vi "FGV_AnalysersControl.vi"(6 "String Input":string, 7 "Action":T2=enum."Get ID", 8 "Error In":errorcluster, 9 "Set Voltage":dbl, 10 "Analyser":i32=1 min=1 max=2 step=1, 11 "VISA resource In":refnum<visa-resource-name>) -> (0 "error out":errorcluster, 2 "Received":string, 3 "VISA resource Out":refnum<visa-resource-name>)   [LabVIEW 2014]
uses:
  TypeDef_AnalyserActions.ctl
panel:
  out "Use Checksum":bool
  in  "Maximum Voltages":T1={"RE"=300.0, "LE"=100.0, "DX"=11.0, "DY"=11.0, "AM"=15.0, "IH"=35.0, "OH"=20.0}
  in  "Minimum Voltages":T1={"RE"=0.0, "LE"=0.0, "DX"=-11.0, "DY"=-11.0, "AM"=0.0, "IH"=5.0, "OH"=5.0}
  # "To update calibration, change the values above\nBE SURE TO CLICK EDIT->MAKE CURRENT VALUES DEFAULT"
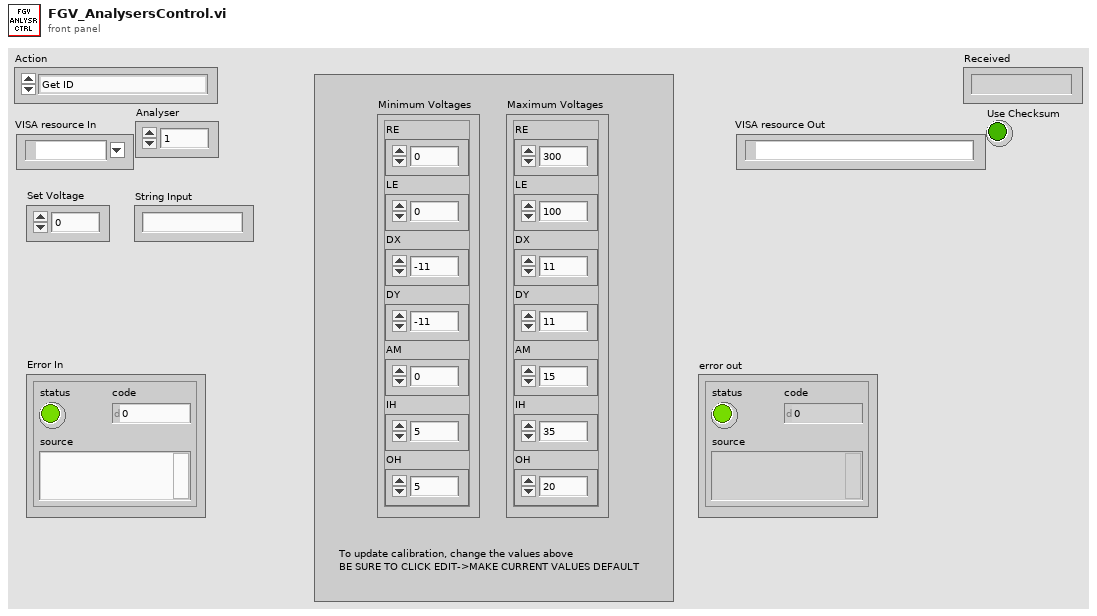
[diagram p1: front panel]
types:
  T1 = cluster{"RE":dbl, "LE":dbl, "DX":dbl, "DY":dbl, "AM":dbl, "IH":dbl, "OH":dbl}
  T2 = typedef "TypeDef_AnalyserActions.ctl" = enum16{"Find COM Port", "Find & Connect", "Connect Port", "Disconnect Port", "Enable Checksum", "Disable Checksum", "Get ID", "Msg & ACKNAK", "Msg & Response", "Set RE Voltage", "Set LE Voltage", "Set DX Voltage", "Set DY Voltage", "Set AM Voltage", "Set IH Voltage", "Set OH Voltage", "Get AE", "Get RE", "Get LE", "Get DX", "Get DY", "Get AM", "Get IH", "Get OH"}
  T3 = cluster{"Maximum Voltages":cluster{"RE":dbl, "LE":dbl, "DX":dbl, "DY":dbl, "AM":dbl, "IH":dbl, "OH":dbl}, "Minimum Voltages":cluster{"RE":dbl, "LE":dbl, "DX":dbl, "DY":dbl, "AM":dbl, "IH":dbl, "OH":dbl}}
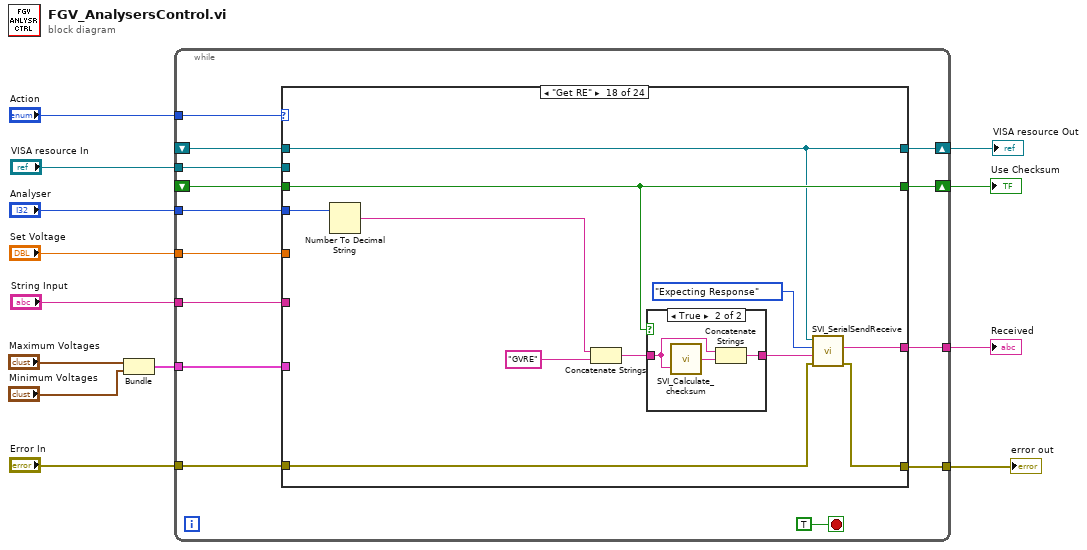
[diagram p0: block diagram]
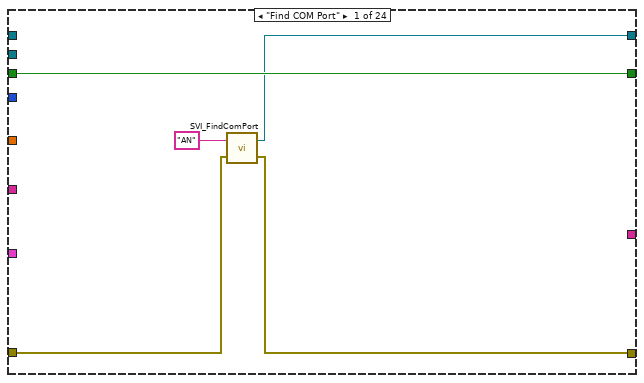
[diagram p2: hidden frame]
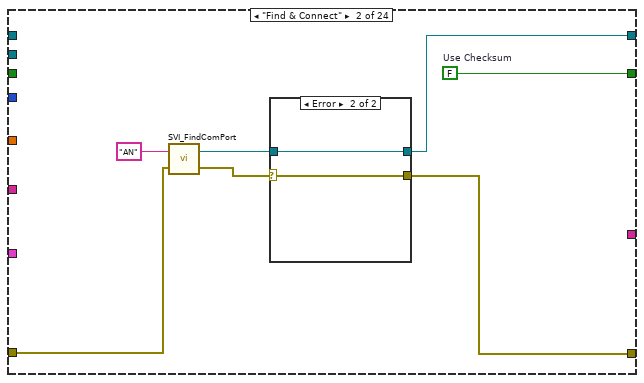
[diagram p3: hidden frame]
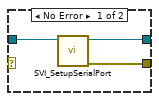
[diagram p4: hidden frame]
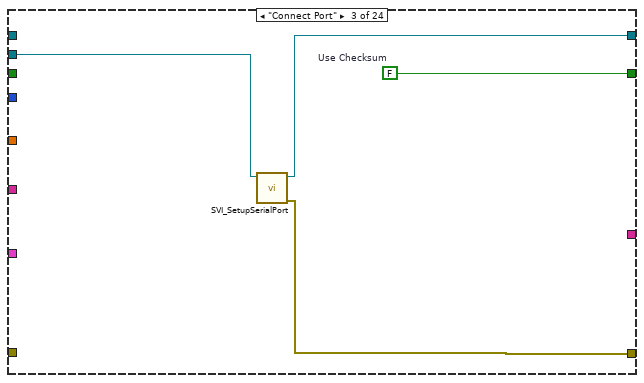
[diagram p5: hidden frame]
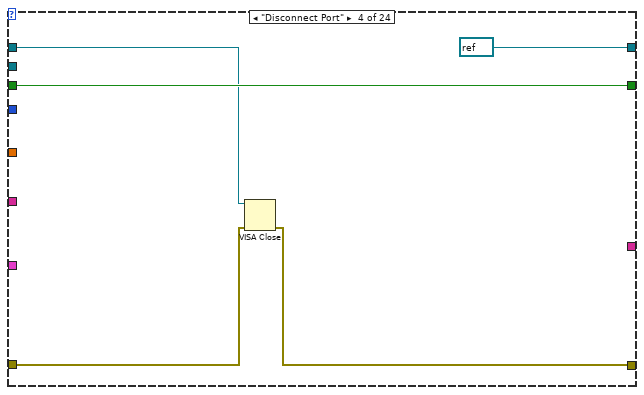
[diagram p6: hidden frame]
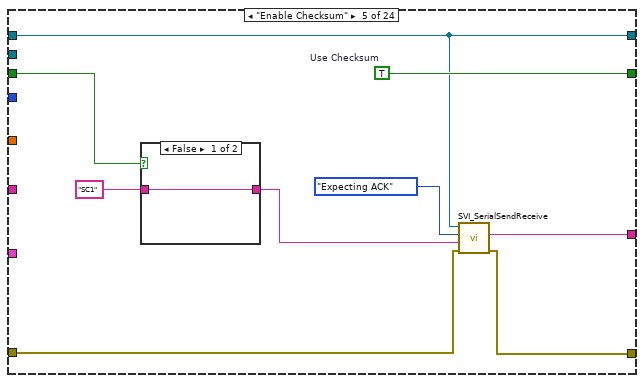
[diagram p7: hidden frame]
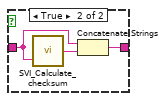
[diagram p8: hidden frame]
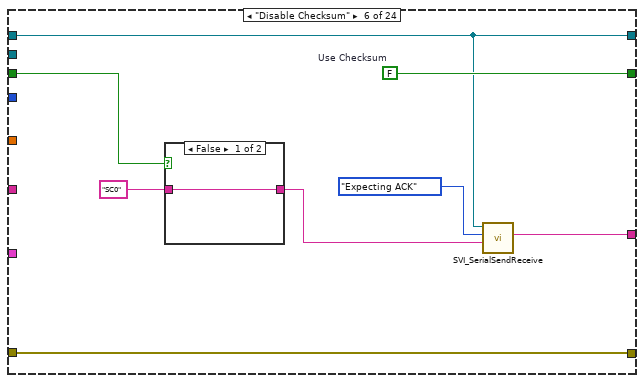
[diagram p9: hidden frame]
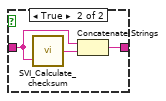
[diagram p10: hidden frame]
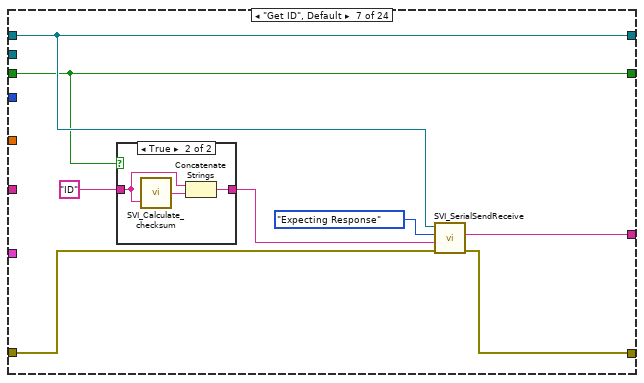
[diagram p11: hidden frame]
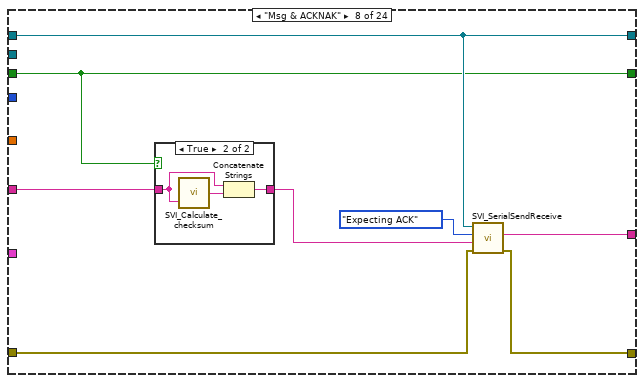
[diagram p13: hidden frame]
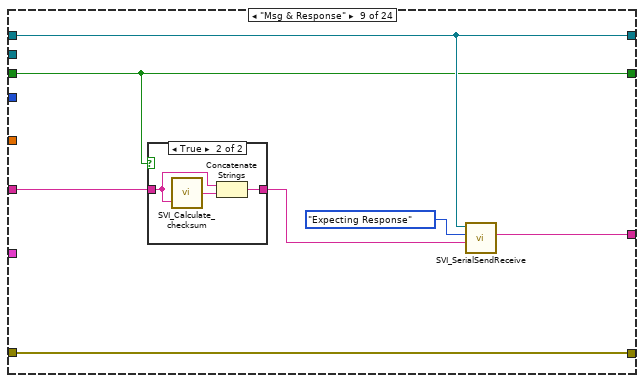
[diagram p15: hidden frame]
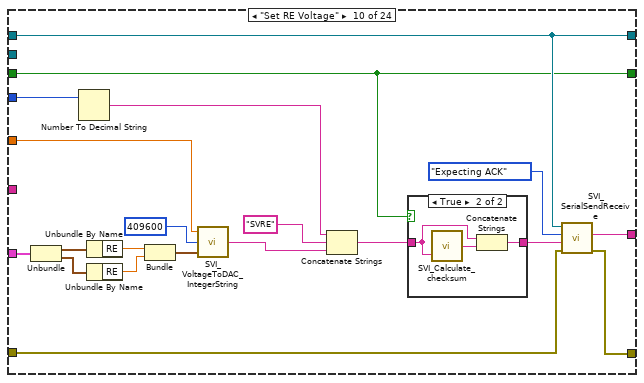
[diagram p17: hidden frame]
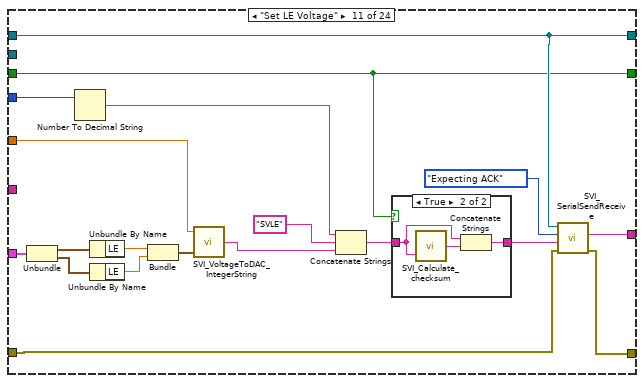
[diagram p19: hidden frame]
diagram:
  n1 = Bundle("Maximum Voltages"="Maximum Voltages", "Minimum Voltages"="Minimum Voltages") -> (w2:T3)  [unwired: 1 in]
  n2 = while {
    tunnel: "Action" -> [w26]
    tunnel: "VISA resource In" -> [w25]
    shift-right: [w24] -> w11
    shift-left: _ -> [w23]
    tunnel: "Error In" -> [w22]
    tunnel: [w21] -> w9
    tunnel: w2 -> [w20]
    tunnel: "Set Voltage" -> [w19]
    shift-right: [w18] -> w6
    shift-left: _ -> [w17]
    tunnel: "String Input" -> [w16]
    tunnel: [w15] -> w7
    tunnel: "Analyser" -> [w14]
    stop <- TRUE stop-if-true
    n3 = case shown="\"Get RE\"" w26 {
      tunnel: w25 -> [_ _ w46 _ _ _ _ _ _ _ _ _ _ _ _ _ _ _ _ _ _ _ _ _]
      tunnel: [w30 w33 w45 refnum<visa-resource-name> refnum ("VISA Refnum out") w57 w67 w83 w95 w105 w130 w147 w163 w188 w213 w230 w254 w279 w293 w306 w324 w338 w353 w369 w381] -> w24
      tunnel: w23 -> [_ _ _ w50 w57 w67 w83 w95 w105 w130 w147 w163 w188 w213 w230 w254 w279 w293 w306 w324 w338 w353 w369 w381]
      tunnel: [w28 w34 w47 w51 w55 w74 w84 w94 w109 w128 w145 w165 w187 w208 w236 w256 w278 w292 w309 w322 w339 w354 w367 w384] -> w21
      tunnel: w22 -> [w29 w37 _ w52 w56 w74 w85 w93 w109 w129 w144 w164 w186 w207 w235 w255 w277 w291 w308 w321 w340 w355 w366 w383]
      tunnel: w20 -> [_ _ _ _ _ _ _ _ _ w121 w149 w166 w184 w211 w234 w258 _ _ _ _ _ _ _ _]
      tunnel: w19 -> [_ _ _ _ _ _ _ _ _ w127 w148 w167 w191 w210 w233 w260 _ _ _ _ _ _ _ _]
      tunnel: [w32 w39 w48 w53 w62 w73 w80 w92 w103 w119 w143 w162 w189 w214 w231 w253 w280 w294 w307 w325 w337 w352 w370 w385] -> w18
      tunnel: w17 -> [w32 _ _ w53 w58 w68 w80 w92 w103 w119 w143 w162 w189 w214 w231 w253 w280 w294 w307 w325 w337 w352 w370 w385]
      tunnel: w16 -> [_ _ _ _ _ _ _ w91 w104 _ _ _ _ _ _ _ _ _ _ _ _ _ _ _]
      tunnel: [_ _ _ _ w54 w69 w79 w96 w106 w131 w146 w161 w185 w212 w237 w257 w276 w296 w310 w323 w341 w356 w368 w382] -> w15
      tunnel: w14 -> [_ _ _ _ _ _ _ _ _ w118 w142 w168 w190 w209 w232 w259 w281 w295 w311 w326 w336 w351 w371 w386]
      frame "Find COM Port" {
        n4 = call "SVI_FindComPort.vi"("Error In"=w29, "ID to Match"="AN") -> ("error out"=w28:errorcluster, "VISA resource name"=w30:refnum<visa-resource-name>)
      }
      frame "Find & Connect" {
        w39 = FALSE  # Use Checksum
        n5 = call "SVI_FindComPort.vi"("Error In"=w37, "ID to Match"="AN") -> ("error out"=w36:errorcluster, "VISA resource name"=w35:refnum<visa-resource-name>)
        n6 = case shown="Error" w36 {
          selector: w36 -> [_ w44]
          tunnel: w35 -> [w42 w43]
          tunnel: [w41 w44] -> w34
          tunnel: [w40 w43] -> w33
          frame No Error {
            n7 = call "SVI_SetupSerialPort.vi"("VISA Refnum in"=w42) -> ("error out"=w41:errorcluster, "VISA Refnum out"=w40:refnum<visa-resource-name>)  [unwired: 9 in]
          }
          frame Error {
          }
        }
      }
      frame "Connect Port" {
        w48 = FALSE  # Use Checksum
        n8 = call "SVI_SetupSerialPort.vi"("VISA Refnum in"=w46) -> ("error out"=w47:errorcluster, "VISA Refnum out"=w45:refnum<visa-resource-name>)  [unwired: 9 in]
      }
      frame "Disconnect Port" {
        n9 = VISA Close(VISA resource name=w50, error in (no error)=w52) -> (error out=w51:errorcluster)
      }
      frame "Enable Checksum" {
        w62 = TRUE  # Use Checksum
        n10 = case shown="False" w58 {
          tunnel: "SC1" ("write buffer") -> [w63 w64]
          tunnel: [w63 w65] -> w60
          frame False {
          }
          frame True {
            n11 = call "SVI_Calculate_checksum.vi"("Message"=w64) -> ("Calculated checksum"=w66:string)  [unwired: 1 in]
            n12 = Concatenate Strings(w64, w66) -> (w65:string)
          }
        }
        n13 = call "SVI_SerialSendReceive.vi"("error in (no error)"=w56, "Command"=w60, "Message Type"=enum16{"Expecting Response", "Expecting ACK"}."Expecting ACK", "VISA Refnum in"=w57) -> ("error out"=w55:errorcluster, "Received"=w54:string)  [unwired: 4 in, 2 out]
      }
      frame "Disable Checksum" {
        w73 = FALSE  # Use Checksum
        n14 = case shown="False" w68 {
          tunnel: "SC0" ("write buffer") -> [w75 w76]
          tunnel: [w75 w77] -> w71
          frame False {
          }
          frame True {
            n15 = call "SVI_Calculate_checksum.vi"("Message"=w76) -> ("Calculated checksum"=w78:string)  [unwired: 1 in]
            n16 = Concatenate Strings(w76, w78) -> (w77:string)
          }
        }
        n17 = call "SVI_SerialSendReceive.vi"("Command"=w71, "Message Type"=enum16{"Expecting Response", "Expecting ACK"}."Expecting ACK", "VISA Refnum in"=w67) -> ("Received"=w69:string)  [unwired: 5 in, 3 out]
      }
      frame "Get ID", Default {
        n18 = case shown="True" w80 {
          tunnel: "ID" ("write buffer") -> [w87 w88]
          tunnel: [w87 w89] -> w82
          frame False {
          }
          frame True {
            n19 = call "SVI_Calculate_checksum.vi"("Message"=w88) -> ("Calculated checksum"=w90:string)  [unwired: 1 in]
            n20 = Concatenate Strings(w88, w90) -> (w89:string)
          }
        }
        n21 = call "SVI_SerialSendReceive.vi"("error in (no error)"=w85, "Command"=w82, "Message Type"=enum16{"Expecting Response", "Expecting ACK"}."Expecting Response", "VISA Refnum in"=w83) -> ("error out"=w84:errorcluster, "Received"=w79:string)  [unwired: 4 in, 2 out]
      }
      frame "Msg & ACKNAK" {
        n22 = case shown="True" w92 {
          tunnel: w91 -> [w99 w100]
          tunnel: [w99 w101] -> w98
          frame False {
          }
          frame True {
            n23 = call "SVI_Calculate_checksum.vi"("Message"=w100) -> ("Calculated checksum"=w102:string)  [unwired: 1 in]
            n24 = Concatenate Strings(w100, w102) -> (w101:string)
          }
        }
        n25 = call "SVI_SerialSendReceive.vi"("error in (no error)"=w93, "Command"=w98, "Message Type"=enum16{"Expecting Response", "Expecting ACK"}."Expecting ACK", "VISA Refnum in"=w95) -> ("error out"=w94:errorcluster, "Received"=w96:string)  [unwired: 4 in, 2 out]
      }
      frame "Msg & Response" {
        n26 = case shown="True" w103 {
          tunnel: w104 -> [w110 w111]
          tunnel: [w110 w112] -> w108
          frame False {
          }
          frame True {
            n27 = call "SVI_Calculate_checksum.vi"("Message"=w111) -> ("Calculated checksum"=w113:string)  [unwired: 1 in]
            n28 = Concatenate Strings(w111, w113) -> (w112:string)
          }
        }
        n29 = call "SVI_SerialSendReceive.vi"("Command"=w108, "Message Type"=enum16{"Expecting Response", "Expecting ACK"}."Expecting Response", "VISA Refnum in"=w105) -> ("Received"=w106:string)  [unwired: 5 in, 3 out]
      }
      frame "Set RE Voltage" {
        n30 = Unbundle(w121) -> ("Maximum Voltages"=w124:T1, "Minimum Voltages"=w125:T1)
        n31 = Number To Decimal String(number=w118) -> (decimal integer string=w115:string)  [unwired: 1 in]
        n32 = Unbundle By Name(w124) -> ("RE"=w123:dbl)
        n33 = Unbundle By Name(w125) -> ("RE"=w122:dbl)
        n34 = Bundle("RE"=w123, "RE"=w122) -> (w120:cluster{"RE":dbl, "RE":dbl})  [unwired: 1 in]
        n35 = call "SVI_VoltageToDAC_IntegerString.vi"("Voltage Limits"=w120, "Divisions (Precision)"=409600, "Set Voltage"=w127) -> ("DAC Int String"=w114:string)
        n36 = Concatenate Strings(w115, "SVRE" ("string"), w114) -> (w116:string)
        n37 = case shown="True" w119 {
          tunnel: w116 -> [w134 w135]
          tunnel: [w134 w136] -> w133
          frame False {
          }
          frame True {
            n38 = call "SVI_Calculate_checksum.vi"("Message"=w135) -> ("Calculated checksum"=w137:string)  [unwired: 1 in]
            n39 = Concatenate Strings(w135, w137) -> (w136:string)
          }
        }
        n40 = call "SVI_SerialSendReceive.vi"("error in (no error)"=w129, "Command"=w133, "Message Type"=enum16{"Expecting Response", "Expecting ACK"}."Expecting ACK", "VISA Refnum in"=w130) -> ("error out"=w128:errorcluster, "Received"=w131:string)  [unwired: 4 in, 2 out]
      }
      frame "Set LE Voltage" {
        n41 = Unbundle(w149) -> ("Maximum Voltages"=w153:T1, "Minimum Voltages"=w154:T1)
        n42 = Number To Decimal String(number=w142) -> (decimal integer string=w140:string)  [unwired: 1 in]
        n43 = Unbundle By Name(w153) -> ("LE"=w152:dbl)
        n44 = Unbundle By Name(w154) -> ("LE"=w151:dbl)
        n45 = Bundle("LE"=w152, "LE"=w151) -> (w150:cluster{"LE":dbl, "LE":dbl})  [unwired: 1 in]
        n46 = call "SVI_VoltageToDAC_IntegerString.vi"("Voltage Limits"=w150, "Set Voltage"=w148) -> ("DAC Int String"=w139:string)  [unwired: 1 in]
        n47 = Concatenate Strings(w140, "SVLE" ("string"), w139) -> (w141:string)
        n48 = case shown="True" w143 {
          tunnel: w141 -> [w157 w158]
          tunnel: [w157 w159] -> w156
          frame False {
          }
          frame True {
            n49 = call "SVI_Calculate_checksum.vi"("Message"=w158) -> ("Calculated checksum"=w160:string)  [unwired: 1 in]
            n50 = Concatenate Strings(w158, w160) -> (w159:string)
          }
        }
        n51 = call "SVI_SerialSendReceive.vi"("error in (no error)"=w144, "Command"=w156, "Message Type"=enum16{"Expecting Response", "Expecting ACK"}."Expecting ACK", "VISA Refnum in"=w147) -> ("error out"=w145:errorcluster, "Received"=w146:string)  [unwired: 4 in, 2 out]
      }
      frame "Set DX Voltage" {
        n52 = Unbundle(w166) -> ("Maximum Voltages"=w176:T1, "Minimum Voltages"=w177:T1)
        n53 = Number To Decimal String(number=w168) -> (decimal integer string=w171:string)  [unwired: 1 in]
        n54 = Unbundle By Name(w176) -> ("DX"=w175:dbl)
        n55 = Unbundle By Name(w177) -> ("DX"=w174:dbl)
        n56 = Bundle("DX"=w175, "DX"=w174) -> (w173:cluster{"DX":dbl, "DX":dbl})  [unwired: 1 in]
        n57 = call "SVI_VoltageToDAC_IntegerString.vi"("Voltage Limits"=w173, "Set Voltage"=w167) -> ("DAC Int String"=w170:string)  [unwired: 1 in]
        n58 = Concatenate Strings(w171, "SVDX" ("string"), w170) -> (w172:string)
        n59 = case shown="True" w162 {
          tunnel: w172 -> [w180 w181]
          tunnel: [w180 w182] -> w179
          frame False {
          }
          frame True {
            n60 = call "SVI_Calculate_checksum.vi"("Message"=w181) -> ("Calculated checksum"=w183:string)  [unwired: 1 in]
            n61 = Concatenate Strings(w181, w183) -> (w182:string)
          }
        }
        n62 = call "SVI_SerialSendReceive.vi"("error in (no error)"=w164, "Command"=w179, "Message Type"=enum16{"Expecting Response", "Expecting ACK"}."Expecting ACK", "VISA Refnum in"=w163) -> ("error out"=w165:errorcluster, "Received"=w161:string)  [unwired: 4 in, 2 out]
      }
      frame "Set DY Voltage" {
        n63 = Unbundle(w184) -> ("Maximum Voltages"=w199:T1, "Minimum Voltages"=w200:T1)
        n64 = Number To Decimal String(number=w190) -> (decimal integer string=w194:string)  [unwired: 1 in]
        n65 = Unbundle By Name(w199) -> ("DY"=w198:dbl)
        n66 = Unbundle By Name(w200) -> ("DY"=w197:dbl)
        n67 = Bundle("DY"=w198, "DY"=w197) -> (w196:cluster{"DY":dbl, "DY":dbl})  [unwired: 1 in]
        n68 = call "SVI_VoltageToDAC_IntegerString.vi"("Voltage Limits"=w196, "Set Voltage"=w191) -> ("DAC Int String"=w193:string)  [unwired: 1 in]
        n69 = Concatenate Strings(w194, "SVDY" ("string"), w193) -> (w195:string)
        n70 = case shown="True" w189 {
          tunnel: w195 -> [w203 w204]
          tunnel: [w203 w205] -> w202
          frame False {
          }
          frame True {
            n71 = call "SVI_Calculate_checksum.vi"("Message"=w204) -> ("Calculated checksum"=w206:string)  [unwired: 1 in]
            n72 = Concatenate Strings(w204, w206) -> (w205:string)
          }
        }
        n73 = call "SVI_SerialSendReceive.vi"("error in (no error)"=w186, "Command"=w202, "Message Type"=enum16{"Expecting Response", "Expecting ACK"}."Expecting ACK", "VISA Refnum in"=w188) -> ("error out"=w187:errorcluster, "Received"=w185:string)  [unwired: 4 in, 2 out]
      }
      frame "Set AM Voltage" {
        n74 = Unbundle(w211) -> ("Maximum Voltages"=w222:T1, "Minimum Voltages"=w223:T1)
        n75 = Number To Decimal String(number=w209) -> (decimal integer string=w217:string)  [unwired: 1 in]
        n76 = Unbundle By Name(w222) -> ("AM"=w221:dbl)
        n77 = Unbundle By Name(w223) -> ("AM"=w220:dbl)
        n78 = Bundle("AM"=w221, "AM"=w220) -> (w219:cluster{"AM":dbl, "AM":dbl})  [unwired: 1 in]
        n79 = call "SVI_VoltageToDAC_IntegerString.vi"("Voltage Limits"=w219, "Set Voltage"=w210) -> ("DAC Int String"=w216:string)  [unwired: 1 in]
        n80 = Concatenate Strings(w217, "SVAM" ("string"), w216) -> (w218:string)
        n81 = case shown="True" w214 {
          tunnel: w218 -> [w226 w227]
          tunnel: [w226 w228] -> w225
          frame False {
          }
          frame True {
            n82 = call "SVI_Calculate_checksum.vi"("Message"=w227) -> ("Calculated checksum"=w229:string)  [unwired: 1 in]
            n83 = Concatenate Strings(w227, w229) -> (w228:string)
          }
        }
        n84 = call "SVI_SerialSendReceive.vi"("error in (no error)"=w207, "Command"=w225, "Message Type"=enum16{"Expecting Response", "Expecting ACK"}."Expecting ACK", "VISA Refnum in"=w213) -> ("error out"=w208:errorcluster, "Received"=w212:string)  [unwired: 4 in, 2 out]
      }
      frame "Set IH Voltage" {
        n85 = Unbundle(w234) -> ("Maximum Voltages"=w245:T1, "Minimum Voltages"=w246:T1)
        n86 = Number To Decimal String(number=w232) -> (decimal integer string=w240:string)  [unwired: 1 in]
        n87 = Unbundle By Name(w245) -> ("IH"=w244:dbl)
        n88 = Unbundle By Name(w246) -> ("IH"=w243:dbl)
        n89 = Bundle("IH"=w244, "IH"=w243) -> (w242:cluster{"IH":dbl, "IH":dbl})  [unwired: 1 in]
        n90 = call "SVI_VoltageToDAC_IntegerString.vi"("Voltage Limits"=w242, "Set Voltage"=w233) -> ("DAC Int String"=w239:string)  [unwired: 1 in]
        n91 = Concatenate Strings(w240, "SVIH" ("string"), w239) -> (w241:string)
        n92 = case shown="True" w231 {
          tunnel: w241 -> [w249 w250]
          tunnel: [w249 w251] -> w248
          frame False {
          }
          frame True {
            n93 = call "SVI_Calculate_checksum.vi"("Message"=w250) -> ("Calculated checksum"=w252:string)  [unwired: 1 in]
            n94 = Concatenate Strings(w250, w252) -> (w251:string)
          }
        }
        n95 = call "SVI_SerialSendReceive.vi"("error in (no error)"=w235, "Command"=w248, "Message Type"=enum16{"Expecting Response", "Expecting ACK"}."Expecting ACK", "VISA Refnum in"=w230) -> ("error out"=w236:errorcluster, "Received"=w237:string)  [unwired: 4 in, 2 out]
      }
      frame "Set OH Voltage" {
        n96 = Unbundle(w258) -> ("Maximum Voltages"=w268:T1, "Minimum Voltages"=w269:T1)
        n97 = Number To Decimal String(number=w259) -> (decimal integer string=w263:string)  [unwired: 1 in]
        n98 = Unbundle By Name(w268) -> ("OH"=w267:dbl)
        n99 = Unbundle By Name(w269) -> ("OH"=w266:dbl)
        n100 = Bundle("OH"=w267, "OH"=w266) -> (w265:cluster{"OH":dbl, "OH":dbl})  [unwired: 1 in]
        n101 = call "SVI_VoltageToDAC_IntegerString.vi"("Voltage Limits"=w265, "Set Voltage"=w260) -> ("DAC Int String"=w262:string)  [unwired: 1 in]
        n102 = Concatenate Strings(w263, "SVOH" ("string"), w262) -> (w264:string)
        n103 = case shown="True" w253 {
          tunnel: w264 -> [w272 w273]
          tunnel: [w272 w274] -> w271
          frame False {
          }
          frame True {
            n104 = call "SVI_Calculate_checksum.vi"("Message"=w273) -> ("Calculated checksum"=w275:string)  [unwired: 1 in]
            n105 = Concatenate Strings(w273, w275) -> (w274:string)
          }
        }
        n106 = call "SVI_SerialSendReceive.vi"("error in (no error)"=w255, "Command"=w271, "Message Type"=enum16{"Expecting Response", "Expecting ACK"}."Expecting ACK", "VISA Refnum in"=w254) -> ("error out"=w256:errorcluster, "Received"=w257:string)  [unwired: 4 in, 2 out]
      }
      frame "Get AE" {
        n107 = Number To Decimal String(number=w281) -> (decimal integer string=w283:string)  [unwired: 1 in]
        n108 = Concatenate Strings(w283, "GVAE" ("string")) -> (w284:string)
        n109 = case shown="True" w280 {
          tunnel: w284 -> [w287 w288]
          tunnel: [w287 w289] -> w286
          frame False {
          }
          frame True {
            n110 = call "SVI_Calculate_checksum.vi"("Message"=w288) -> ("Calculated checksum"=w290:string)  [unwired: 1 in]
            n111 = Concatenate Strings(w288, w290) -> (w289:string)
          }
        }
        n112 = call "SVI_SerialSendReceive.vi"("error in (no error)"=w277, "Command"=w286, "Message Type"=enum16{"Expecting Response", "Expecting ACK"}."Expecting Response", "VISA Refnum in"=w279) -> ("error out"=w278:errorcluster, "Received"=w276:string)  [unwired: 4 in, 2 out]
      }
      frame "Get RE" {
        n113 = Number To Decimal String(number=w295) -> (decimal integer string=w298:string)  [unwired: 1 in]
        n114 = Concatenate Strings(w298, "GVRE" ("string")) -> (w299:string)
        n115 = case shown="True" w294 {
          tunnel: w299 -> [w302 w303]
          tunnel: [w302 w304] -> w301
          frame False {
          }
          frame True {
            n116 = call "SVI_Calculate_checksum.vi"("Message"=w303) -> ("Calculated checksum"=w305:string)  [unwired: 1 in]
            n117 = Concatenate Strings(w303, w305) -> (w304:string)
          }
        }
        n118 = call "SVI_SerialSendReceive.vi"("error in (no error)"=w291, "Command"=w301, "Message Type"=enum16{"Expecting Response", "Expecting ACK"}."Expecting Response", "VISA Refnum in"=w293) -> ("error out"=w292:errorcluster, "Received"=w296:string)  [unwired: 4 in, 2 out]
      }
      frame "Get LE" {
        n119 = Number To Decimal String(number=w311) -> (decimal integer string=w313:string)  [unwired: 1 in]
        n120 = Concatenate Strings(w313, "GVLE" ("string")) -> (w314:string)
        n121 = case shown="True" w307 {
          tunnel: w314 -> [w317 w318]
          tunnel: [w317 w319] -> w316
          frame False {
          }
          frame True {
            n122 = call "SVI_Calculate_checksum.vi"("Message"=w318) -> ("Calculated checksum"=w320:string)  [unwired: 1 in]
            n123 = Concatenate Strings(w318, w320) -> (w319:string)
          }
        }
        n124 = call "SVI_SerialSendReceive.vi"("error in (no error)"=w308, "Command"=w316, "Message Type"=enum16{"Expecting Response", "Expecting ACK"}."Expecting Response", "VISA Refnum in"=w306) -> ("error out"=w309:errorcluster, "Received"=w310:string)  [unwired: 4 in, 2 out]
      }
      frame "Get DX" {
        n125 = Number To Decimal String(number=w326) -> (decimal integer string=w328:string)  [unwired: 1 in]
        n126 = Concatenate Strings(w328, "GVDX" ("string")) -> (w329:string)
        n127 = case shown="True" w325 {
          tunnel: w329 -> [w332 w333]
          tunnel: [w332 w334] -> w331
          frame False {
          }
          frame True {
            n128 = call "SVI_Calculate_checksum.vi"("Message"=w333) -> ("Calculated checksum"=w335:string)  [unwired: 1 in]
            n129 = Concatenate Strings(w333, w335) -> (w334:string)
          }
        }
        n130 = call "SVI_SerialSendReceive.vi"("error in (no error)"=w321, "Command"=w331, "Message Type"=enum16{"Expecting Response", "Expecting ACK"}."Expecting Response", "VISA Refnum in"=w324) -> ("error out"=w322:errorcluster, "Received"=w323:string)  [unwired: 4 in, 2 out]
      }
      frame "Get DY" {
        n131 = Number To Decimal String(number=w336) -> (decimal integer string=w343:string)  [unwired: 1 in]
        n132 = Concatenate Strings(w343, "GVDY" ("string")) -> (w344:string)
        n133 = case shown="True" w337 {
          tunnel: w344 -> [w347 w348]
          tunnel: [w347 w349] -> w346
          frame False {
          }
          frame True {
            n134 = call "SVI_Calculate_checksum.vi"("Message"=w348) -> ("Calculated checksum"=w350:string)  [unwired: 1 in]
            n135 = Concatenate Strings(w348, w350) -> (w349:string)
          }
        }
        n136 = call "SVI_SerialSendReceive.vi"("error in (no error)"=w340, "Command"=w346, "Message Type"=enum16{"Expecting Response", "Expecting ACK"}."Expecting Response", "VISA Refnum in"=w338) -> ("error out"=w339:errorcluster, "Received"=w341:string)  [unwired: 4 in, 2 out]
      }
      frame "Get AM" {
        n137 = Number To Decimal String(number=w351) -> (decimal integer string=w358:string)  [unwired: 1 in]
        n138 = Concatenate Strings(w358, "GVAM" ("string")) -> (w359:string)
        n139 = case shown="True" w352 {
          tunnel: w359 -> [w362 w363]
          tunnel: [w362 w364] -> w361
          frame False {
          }
          frame True {
            n140 = call "SVI_Calculate_checksum.vi"("Message"=w363) -> ("Calculated checksum"=w365:string)  [unwired: 1 in]
            n141 = Concatenate Strings(w363, w365) -> (w364:string)
          }
        }
        n142 = call "SVI_SerialSendReceive.vi"("error in (no error)"=w355, "Command"=w361, "Message Type"=enum16{"Expecting Response", "Expecting ACK"}."Expecting Response", "VISA Refnum in"=w353) -> ("error out"=w354:errorcluster, "Received"=w356:string)  [unwired: 4 in, 2 out]
      }
      frame "Get IH" {
        n143 = Number To Decimal String(number=w371) -> (decimal integer string=w373:string)  [unwired: 1 in]
        n144 = Concatenate Strings(w373, "GVIH" ("string")) -> (w374:string)
        n145 = case shown="True" w370 {
          tunnel: w374 -> [w377 w378]
          tunnel: [w377 w379] -> w376
          frame False {
          }
          frame True {
            n146 = call "SVI_Calculate_checksum.vi"("Message"=w378) -> ("Calculated checksum"=w380:string)  [unwired: 1 in]
            n147 = Concatenate Strings(w378, w380) -> (w379:string)
          }
        }
        n148 = call "SVI_SerialSendReceive.vi"("error in (no error)"=w366, "Command"=w376, "Message Type"=enum16{"Expecting Response", "Expecting ACK"}."Expecting Response", "VISA Refnum in"=w369) -> ("error out"=w367:errorcluster, "Received"=w368:string)  [unwired: 4 in, 2 out]
      }
      frame "Get OH" {
        n149 = Number To Decimal String(number=w386) -> (decimal integer string=w388:string)  [unwired: 1 in]
        n150 = Concatenate Strings(w388, "GVOH" ("string")) -> (w389:string)
        n151 = case shown="True" w385 {
          tunnel: w389 -> [w392 w393]
          tunnel: [w392 w394] -> w391
          frame False {
          }
          frame True {
            n152 = call "SVI_Calculate_checksum.vi"("Message"=w393) -> ("Calculated checksum"=w395:string)  [unwired: 1 in]
            n153 = Concatenate Strings(w393, w395) -> (w394:string)
          }
        }
        n154 = call "SVI_SerialSendReceive.vi"("error in (no error)"=w383, "Command"=w391, "Message Type"=enum16{"Expecting Response", "Expecting ACK"}."Expecting Response", "VISA Refnum in"=w381) -> ("error out"=w384:errorcluster, "Received"=w382:string)  [unwired: 4 in, 2 out]
      }
    }
  }
  "VISA resource Out" <- w11
  "error out" <- w9
  "Received" <- w7
  "Use Checksum" <- w6
